vi "Read GUI Events.vi"(8 "error in (no error)":errorcluster, 11 "CS++SVMonitor in":refnum<class "CS++SVMonitor.lvclass">) -> (0 "error out":errorcluster, 2 "GUI Events":T1, 3 "CS++SVMonitor out":refnum<class "CS++SVMonitor.lvclass">)   [LabVIEW 2016, in "CS++SVMonitor.lvlib" / "CS++SVMonitor.lvclass"]
doc: "Read GUI event references from attribute."
uses:
  CS++SVMonitor.lvclass
  <vilib>/ActorFramework/Message Enqueuer/Message Enqueuer.lvclass
  CS++PVMonitor Messages/CS++PVUpdate Msg/CS++PVUpdate Msg.lvclass
  CS++SVMonitor.lvclass/CS++SVMonitor.ctl
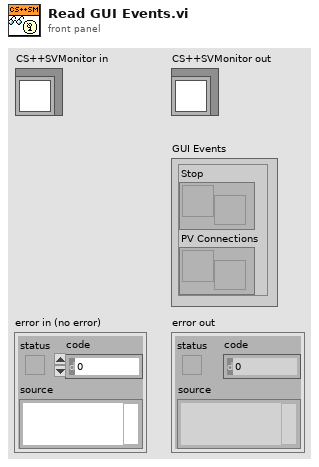
[diagram p1: front panel]
types:
  T1 = cluster{"Stop":refnum<user-event>, "PV Connections":refnum<user-event>}
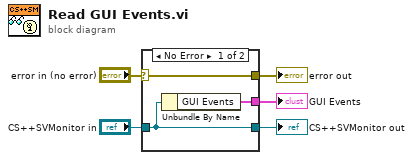
[diagram p0: block diagram]
diagram:
  n1 = case shown="No Error" "error in (no error)" {
    selector: "error in (no error)" -> [w8 w9]
    tunnel: [w8 w9] -> w4
    tunnel: [w7 w10] -> w2
    tunnel: "CS++SVMonitor in" -> [w7 w10]
    tunnel: [w6 _] -> w1
    frame No Error {
      n2 = Unbundle By Name(w7) -> ("GUI Events"=w6:T1)
    }
    frame Error {
    }
  }
  "error out" <- w4
  "CS++SVMonitor out" <- w2
  "GUI Events" <- w1
